vi "PH_PSDBController.get Experiments.vi"(0 "i ref in":refnum<vi>, 2 "possible Experiments":T1[](array[typedef]), 5 "error IO":errorcluster) -> (14 "i ref out":refnum<vi>, 19 "error out":errorcluster)   [LabVIEW 2014, in "PH_PSDBController.lvlib"]
doc: "This VI sets the incoming possible experiments to own atributes, publishes them as DIM service and sets related to that the current experiment."
uses:
  PH_PSDBController.lvlib
  CSlibraries-extern/psdb_lv/PSDB_Info.ctl
  CSlibraries/UtilityLib/UtilityLib.lvlib
  CS_Core/CSSystem/CoreLib/CoreLib.lvlib
  CSlibraries-extern/DimLVEvent/LVDimInterface/LVDimInterface.lvlib
  CSlibraries-extern/psdb_lv/PSDB.lvlib
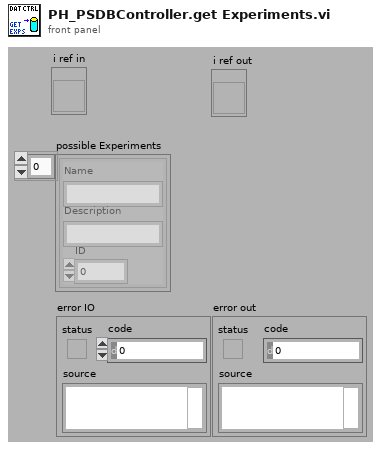
[diagram p1: front panel]
types:
  T1 = typedef "PSDB.lvlib/PSDB_Info.ctl" = cluster{"Name":string, "Description":string, "ID":i32}
  T2 = typedef "PH_PSDBController.lvlib/PH_PSDBController.i attribute.ctl" = cluster{"GUI Refs":cluster{"Data Status":refnum<vi>, "Current Shot ID":refnum<vi>, "active Subsystems":refnum<vi>, "Experiment Description":refnum<vi>, "Shot Comment":refnum<vi>, "Experiment":refnum<vi>, "Shottype":refnum<vi>, "Sequencer SM State":refnum<vi>, "Instances with Errors":refnum<vi>}, "Service ID Shot ID":i32, "Service ID wanted Subsystem":i32, "Data Status":T3, "Shotinformation":cluster{"Current Experiment ID":i32, "Current Shot Type":i32, "Current Comment":string}, "Data taking?":bool, "Service ID current Shottype":i32, "Service ID current Experiment":i32, "Service ID currentShot Comment":i32, "Service ID possible Shottypes":i32, "Service ID possible Experiments":i32, "possible Experiments":T1[], "possible Shottypes":T1[], "List":cluster{"Info":cluster{"Instance":string, "Data Status":T3}[], "GUI Ref":refnum<vi>, "Classname":string}[], "Subsystems Off?":cluster{"PHELIX_Beamline_fs_YLF_BL_Status":bool, "PHELIX_Beamline_ns_BL_Status":bool, "PHELIX_Beamline_PA_Input_BL_Status":bool, "PHELIX_Beamline_PA_MA_BL_Status":bool, "PHELIX_Beamline_MA_Z6_BL_Status":bool, "PHELIX_Beamline_MA_LB_BL_Status":bool, "PHELIX_Beamline_PA_LL_BL_Status":bool}, "PSDB Credentials":T4}
  T3 = typedef "PH_PSDBWriter.lvlib/PH_PSDBWriter.Data Status.ctl" = i16
  T4 = typedef "PH_Common.lvlib/PH_Connection.PSDB Credentials.ctl" = cluster{"PW":string, "ID":string, "DS":string}
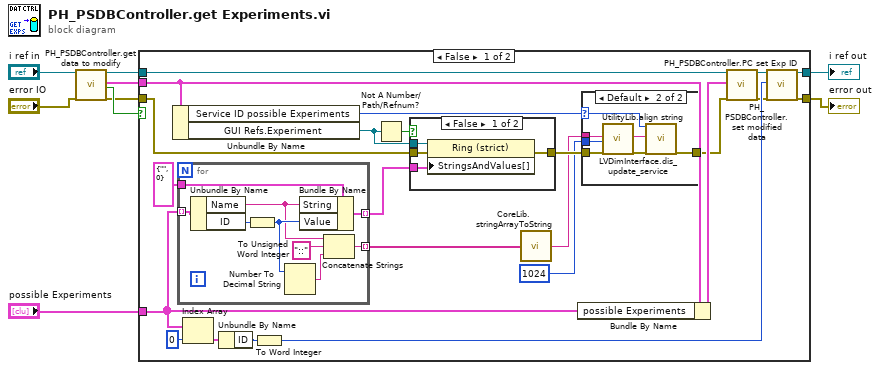
[diagram p0: block diagram]
diagram:
  n1 = call "PH_PSDBController.get data to modify.vi"("i ref in"="i ref in", "error in (no error)"="error IO") -> ("i ref out"=w4:refnum<vi>, "i attribute"=w3:T2, "timed out"=w9:bool, "error out"=w5:errorcluster)  [unwired: 14 in]
  n2 = case shown="False" w9 {
    tunnel: w3 -> [w23 _]
    tunnel: w4 -> [w15 w56]
    tunnel: w5 -> [w13 w55]
    tunnel: "possible Experiments" -> [w19 _]
    tunnel: [w26 w56] -> w7
    tunnel: [w24 w55] -> w8
    frame False {
      n3 = Unbundle By Name(w23) -> ("Service ID possible Experiments"=w10:i32, "GUI Refs.Experiment"=w14:refnum<vi>)
      n4 = for {
        tunnel: w19 -> [w54] mode=indexing
        tunnel: [w52] -> w20 mode=indexing
        tunnel: cluster{"String":string, "Value":u16} {"String"="", "Value"=0} -> [w51]
        tunnel: [w46] -> w18 mode=indexing
        n5 = Unbundle By Name(w54) -> ("Name"=w49:string, "ID"=w53:i32)
        n6 = To Unsigned Word Integer(number=w53) -> (unsigned 16bit integer=w50:u16)
        n7 = Number To Decimal String(number=w50) -> (decimal integer string=w47:string)  [unwired: 1 in]
        n8 = Bundle By Name(cluster=w51, "String"=w49, "Value"=w50) -> (w52:cluster{"String":string, "Value":u16})
        n9 = Concatenate Strings(w49, "::" ("string"), w47) -> (w46:string)
      }
      n10 = Index Array(array=w19, index=0 ("Exp ID")) -> (element=w31:T1)
      n11 = Unbundle By Name(w31) -> ("ID"=w30:i32)
      n12 = To Word Integer(number=w30) -> (16bit integer=w28:i16)
      n13 = Not A Number/Path/Refnum?(number/path/refnum=w14) -> (NaN/Path/Refnum?=w21:bool)
      n14 = case shown="False" w21 {
        tunnel: w13 -> [w44 w45]
        tunnel: [w43 w45] -> w17
        tunnel: w14 -> [w42 _]
        tunnel: w20 -> [w41 _]
        frame False {
          n15 = property class="Ring (strict)"(reference=w42, error in=w44, "StringsAndValues[]"=w41) -> (error out=w43:errorcluster)  [unwired: 1 out]
        }
        frame True {
        }
      }
      n16 = call "CoreLib.stringArrayToString.vi"("Array"=w18) -> ("String"=w16:string)
      n17 = Bundle By Name(cluster=w23, "possible Experiments"=w19) -> (w29:T2)
      n18 = case shown="Default" w10 {
        selector: w10 -> [_ w34]
        tunnel: w17 -> [w33 w40]
        tunnel: w16 -> [_ w39]
        tunnel: u16 1024 ("stringLength (80)") -> [_ w38]
        tunnel: [w33 w36] -> w11
        frame -1 {
        }
        frame Default {
          n19 = call "UtilityLib.align string.vi"("stringIn"=w39, "stringLength (80)"=w38, "error in (no error)"=w40) -> ("stringOut"=w35:string, "error out"=w37:errorcluster)  [unwired: 15 in]
          n20 = call "LVDimInterface.dis_update_service.vi"("my_serviceID"=w34, "data"=w35, "error in (no error)"=w37) -> ("error out"=w36:errorcluster)  [unwired: 14 in, 2 out]
        }
      }
      n21 = call "PH_PSDBController.set modified data.vi"("i ref in"=w15, "i attribute"=w29, "error in (no error)"=w11) -> ("i ref out"=w27:refnum<vi>, "error out"=w25:errorcluster)  [unwired: 15 in]
      n22 = call "PH_PSDBController.PC set Exp ID.vi"("i ref in"=w27, "Exp ID"=w28, "error IO"=w25) -> ("i ref out"=w26:refnum<vi>, "error out"=w24:errorcluster)  [unwired: 15 in]
    }
    frame True {
    }
  }
  "error out" <- w8
  "i ref out" <- w7
